vi "SailControlFunction logic demo.vi"() -> ()   [LabVIEW 2011]
doc: "demonstrates the working logic behind the SailControlFunction with linear and trigonometric functions."
panel:
  out "Waveform Graph 3":dbl[](graph)
  in  "Sails Full Out Point":dbl=45.0
  out "Waveform Graph 2":dbl[](graph)
  in  "Sails Full In Point":dbl=45.0
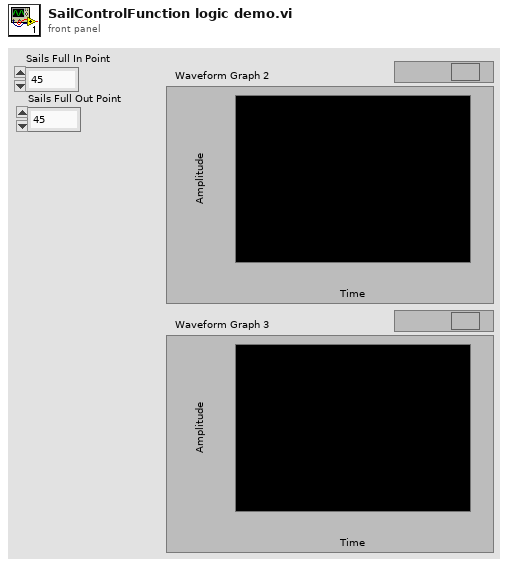
[diagram p1: front panel]
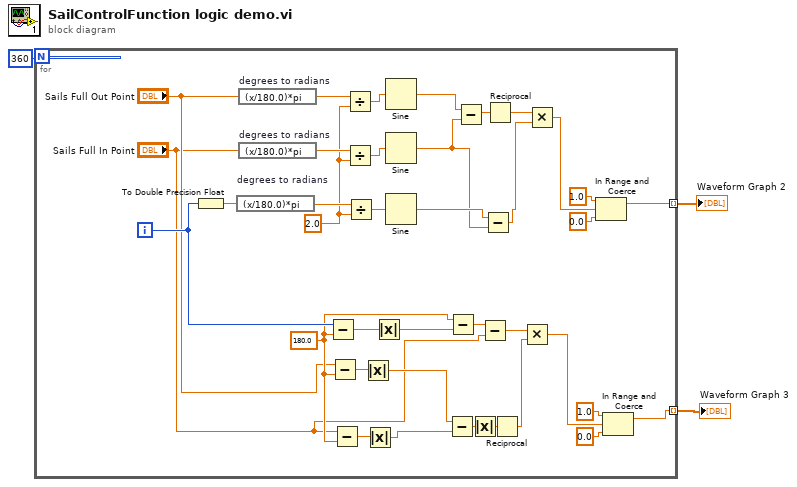
[diagram p0: block diagram]
diagram:
  n1 = for {
    N: 360 -> [_]
    tunnel: [w35] -> w2 mode=indexing
    tunnel: [w19] -> w1 mode=indexing
    i -> [w22]
    w10 = 180.0 ("upper limit")
    w23 = 2.0 ("x")
    n2 = To Double Precision Float(number=w22) -> (double precision float=w38:dbl)
    n3 = expression code="(x/180.0)*pi" "degrees to radians"(w38) -> (w40:dbl)
    n4 = expression code="(x/180.0)*pi" "degrees to radians"("Sails Full Out Point") -> (w30:dbl)
    n5 = expression code="(x/180.0)*pi" "degrees to radians"("Sails Full In Point") -> (w33:dbl)
    n6 = Subtract(x=w22, y=w10) -> (x-y=w18:dbl)
    n7 = Subtract(x="Sails Full Out Point", y=w10) -> (x-y=w17:dbl)
    n8 = Subtract(x="Sails Full In Point", y=w10) -> (x-y=w16:dbl)
    n9 = Divide(x=w30, y=w23) -> (x/y=w31:dbl)
    n10 = Divide(x=w33, y=w23) -> (x/y=w32:dbl)
    n11 = Divide(x=w40, y=w23) -> (x/y=w39:dbl)
    n12 = Absolute Value(x=w17) -> (abs(x)=w6:dbl)
    n13 = Absolute Value(x=w16) -> (abs(x)=w7:dbl)
    n14 = Absolute Value(x=w18) -> (abs(x)=w14:dbl)
    n15 = Sine(x=w31) -> (sin(x)=w29:dbl)
    n16 = Sine(x=w32) -> (sin(x)=w28:dbl)
    n17 = Sine(x=w39) -> (sin(x)=w34:dbl)
    n18 = Subtract(x=w6, y=w7) -> (x-y=w15:dbl)
    n19 = Subtract(x=w10, y=w14) -> (x-y=w9:dbl)
    n20 = Subtract(x=w29, y=w28) -> (x-y=w27:dbl)
    n21 = Absolute Value(x=w15) -> (abs(x)=w11:dbl)
    n22 = Subtract(x=w9, y="Sails Full In Point") -> (x-y=w8:dbl)
    n23 = Subtract(x=w34, y=w28) -> (x-y=w25:dbl)
    n24 = Reciprocal(x=w27) -> (1/x=w26:dbl)
    n25 = Reciprocal(x=w11) -> (1/x=w13:dbl)
    n26 = Multiply(x=w8, y=w13) -> (x*y=w12:dbl)
    n27 = Multiply(x=w26, y=w25) -> (x*y=w24:dbl)
    n28 = In Range and Coerce(upper limit=1.0, x=w24, lower limit=0.0 ("upper limit")) -> (coerced(x)=w35:dbl)  [unwired: 1 out]
    n29 = In Range and Coerce(upper limit=1.0, x=w12, lower limit=0.0 ("upper limit")) -> (coerced(x)=w19:dbl)  [unwired: 1 out]
  }
  "Waveform Graph 2" <- w2
  "Waveform Graph 3" <- w1
